vi "DAQmx Timing (Implicit).vi"(0 "task/channels in":refnum<k21>, 1 "sample mode":i32(ring)=10178 items=["Finite Samples"=10178, "Continuous Samples"=10123, "Hardware Timed Single Point"=12522], 2 "samples per channel":i32=1000, 11 "error in":errorcluster) -> (4 "task out":refnum<k21>, 15 "error out":errorcluster)   [LabVIEW 2020]
doc: "Sets only the number of samples to acquire or generate without specifying timing. Typically, you should use this instance when the task does not require sample timing, such as tasks that use counters for buffered frequency measurement, buffered period measurement, or pulse train generation. For finite counter output tasks, <B>samples per channel</B> is the number of pulses to generate."
uses:
  nilvaiu.dll
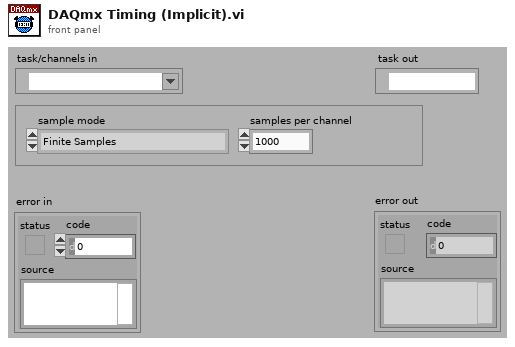
[diagram p1: front panel]
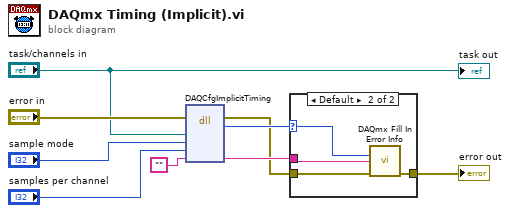
[diagram p0: block diagram]
diagram:
  n1 = dll-call lib="nilvaiu.*" fn="DAQCfgImplicitTiming"(error in="error in", "taskID"="task/channels in", "sampleMode"="sample mode", "samplesPerChannel"="samples per channel", "extendedErrorInfo"="") -> (error out=w1:errorcluster, "return type"=w6:i32, "extendedErrorInfo"=w5:string)  [unwired: 2 in, 4 out]
  n2 = case shown="Default" w6 {
    selector: w6 -> [_ w12]
    tunnel: w1 -> [w10 w14]
    tunnel: [w10 w13] -> w9
    tunnel: w5 -> [_ w11]
    frame 0 {
    }
    frame Default {
      n3 = call "DAQmx Fill In Error Info.vi"("status code"=w12, "extended error info"=w11, "error in"=w14) -> ("error out"=w13:errorcluster)  [unwired: 1 in, 11 out]
    }
  }
  "error out" <- w9
  "task out" <- "task/channels in"
